vi "Cube identification.vi"(7 "error in":errorcluster) -> (27 "error out":errorcluster)   [LabVIEW 2020]
uses:
  <vilib>/vision/NI_Vision_Development_Module.lvlib
panel:
  out "Image Out":T1(plugin-control)
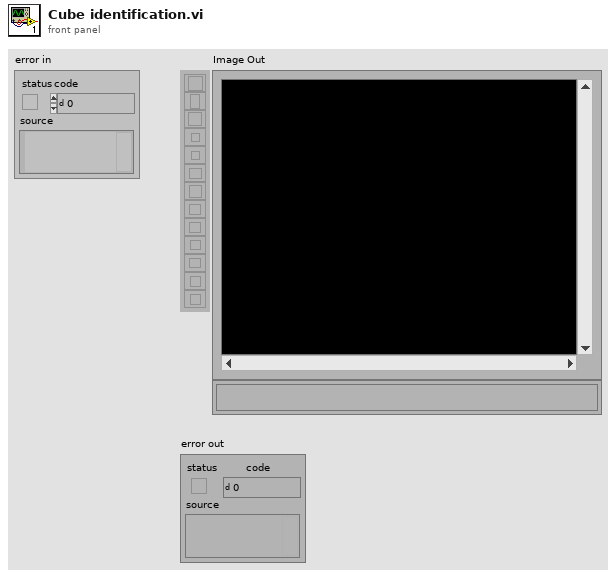
[diagram p1: front panel]
types:
  T1 = typedef "IMAQ Image.ctl" = refnum<image>
  T2 = typedef "Image Type" = u32
  T3 = cluster{"Global Rectangle":i32[], "Contours":cluster{"ID":enum32{"External", "Internal"}, "Type":u32, "Coordinates":i32[]}[]}
  T4 = cluster{"Position":cluster{"x":sgl, "y":sgl}, "Angle":sgl, "Scale":sgl, "Score":sgl, "Bounding Box":cluster{"x":sgl, "y":sgl}[]}[]
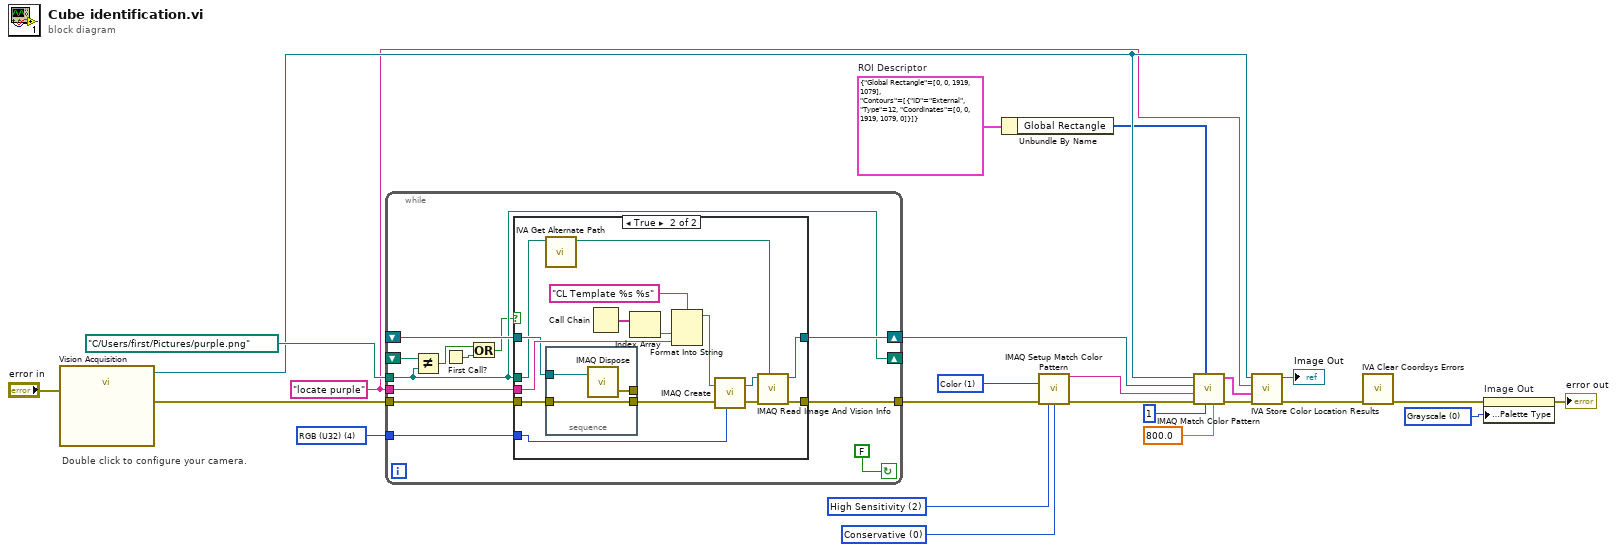
[diagram p0: block diagram]
diagram:
  w1 = u32 0 items=["Grayscale", "Binary", "Gradient", "Rainbow", "Temperature", "User Defined", "Binary 16 Bit", "Gradient 16 Bit", "Rainbow 16 Bit", "Temperature 16 Bit", "User Defined 16 Bit"] ("Palette Type")
  w11 = "locate purple" ("Step Name")
  w17 = T2 4 items=["Grayscale (U8)", "Grayscale (I16)", "Grayscale (SGL)", "Complex (CSG)", "RGB (U32)", "HSL (U32)", "RGB (U64)"] ("Image Type")
  w19 = u32 0 items=["Conservative", "Balance", "Aggressive", "Very Aggressive"] ("Search Strategy")
  w20 = u32 2 items=["Low Sensitivity", "Medium Sensitivity", "High Sensitivity"] ("Color Sensitivity")
  w21 = u32 1 items=["Color and Shape", "Color", "Shape"] ("Match Feature Mode")
  w16 = T3 {"Global Rectangle"=[0, 0, 1919, 1079], "Contours"=[{"ID"=enum."External", "Type"=12, "Coordinates"=[0, 0, 1919, 1079, 0]}]}  # ROI Descriptor
  # "Double click to configure your camera."
  n1 = call "Vision Acquisition"("error in"="error in") -> ("Image Out"=w13:T1, "error out"=w15:errorcluster)  [unwired: 25 in]
  n2 = while {
    shift-right: [w36] -> w7
    shift-left: _ -> [w35]
    tunnel: [w33] -> w6
    tunnel: w15 -> [w32]
    tunnel: path "C:/Users/first/Pictures/purple.png" ("File Path") -> [w28]
    tunnel: w17 -> [w31]
    tunnel: w11 -> [w30]
    shift-right: [w28] -> _
    shift-left: _ -> [w29]
    stop <- FALSE continue-if-true
    n3 = Not Equal?(x=w29, y=w28) -> (x != y?=w26:bool)
    n4 = First Call?() -> (First Call?: T/F=w27:bool)
    n5 = Or(x=w26, y=w27) -> (x .or. y?=w25:bool)
    n6 = case shown="True" w25 {
      tunnel: [w38 w51] -> w36
      tunnel: w35 -> [w38 w43]
      tunnel: [w37 w48] -> w33
      tunnel: w32 -> [w37 w42]
      tunnel: w31 -> [_ w47]
      tunnel: w30 -> [_ w44]
      tunnel: w28 -> [_ w40]
      frame False {
      }
      frame True {
        n7 = call <vilib>:"IVA Get Alternate Path.vi"("Path In"=w40) -> ("Path Out"=w39:path)  [unwired: 10 out]
        n8 = stacked-sequence {
          tunnel: w43 -> [w56]
          tunnel: w42 -> [w55]
          tunnel: [w55] -> w41
          tunnel: [w54] -> _
          frame #0 {
            n9 = call "IMAQ Dispose"("Image"=w56) -> ("error out"=w54:errorcluster)  [unwired: 2 in, 3 out]
          }
        }
        n10 = Call Chain() -> (call chain=w46:string[])
        n11 = Index Array(array=w46) -> (element=w45:string)  [unwired: 1 in]
        n12 = Format Into String(format string="CL Template %s %s" ("Image Name"), w45, w44) -> (resulting string=w53:string)  [unwired: 2 in, 1 out]
        n13 = call "IMAQ Create"("Image Name"=w53, "Image Type"=w47, "error in (no error)"=w41) -> ("New Image"=w50:T1, "error out"=w49:errorcluster)  [unwired: 1 in, 1 out]
        n14 = call "IMAQ Read Image And Vision Info"("File Path"=w39, "error in (no error)"=w49, "Image"=w50) -> ("error out"=w48:errorcluster, "Image Out"=w51:T1)  [unwired: 1 in, 6 out]
      }
    }
  }
  n15 = Unbundle By Name(w16) -> ("Global Rectangle"=w8:i32[])
  n16 = call "IMAQ Setup Match Color Pattern"("Match Feature Mode"=w21, "error in (no error)"=w6, "Color Sensitivity"=w20, "Search Strategy"=w19) -> ("Match Color Pattern Setup Data"=w10:string, "error out"=w9:errorcluster)  [unwired: 5 in, 5 out]
  n17 = call "IMAQ Match Color Pattern"("Minimum Match Score"=sgl 800.0, "Number of Matches Requested"=1, "Optional Rectangle"=w8, "error in (no error)"=w9, "Match Color Pattern Setup Data"=w10, "Template Image"=w7, "Image"=w13) -> ("error out"=w14:errorcluster, "Matches"=w12:T4)  [unwired: 3 out]
  n18 = call <vilib>:"IVA Store Color Location Results.vi"("error in (no error)"=w14, "Matches"=w12, "Step Name"=w11, "Image in"=w13) -> ("error out"=w5:errorcluster, "Image dup"=→"Image Out":T1)  [unwired: 6 out]
  n19 = call <vilib>:"IVA Clear Coordsys Errors.vi"("error in (no error)"=w5) -> ("error out"=w4:errorcluster)  [unwired: 10 in]
  n20 = property on="Image Out" class="ImageControl"(error in=w4, "Palette:Palette Type"=w1) -> (error out=→"error out":errorcluster)  [unwired: 1 in, 1 out]
